vi "Initialize SPI Engine Resources.vi"   [LabVIEW 2015, in "SPI API.lvlib"]
uses:
  SPI API.lvlib
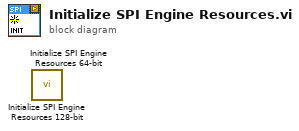
[diagram p0: block diagram]
diagram:
  n1 = call "Initialize SPI Engine Resources 128-bit.vi"() -> ()  [unwired: 10 in, 2 out]
  n2 = call "Initialize SPI Engine Resources 64-bit.vi"() -> ()  [unwired: 10 in, 2 out]
